vi "SB_OUT.vi"(8 "error in (no error)":errorcluster, 10 "拍攝B讀取條碼":string, 11 "DBLink":string) -> (0 "error out":errorcluster, 2 "待出料":cluster{"條碼A":string, "條碼B":string}, 3 "Workspace: screw_B":cluster{"條碼A":string, "條碼B":string}[](array[cluster]))   [LabVIEW 2019]
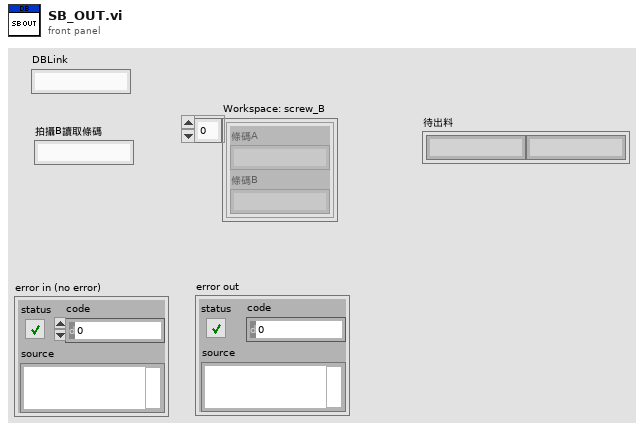
[diagram p1: front panel]
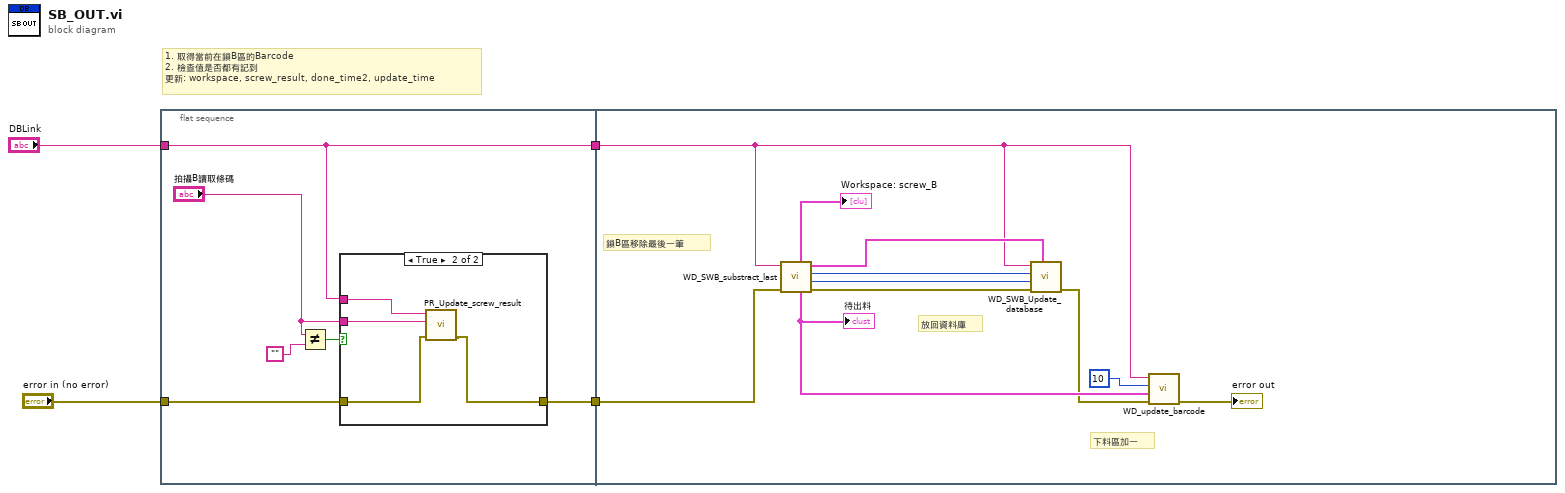
[diagram p0: block diagram]
diagram:
  # "1. 取得當前在鎖B區的Barcode\n2. 檢查值是否都有記到\n更新: workspace, screw_result, done_time2, update_time"
  n1 = flat-sequence {
    tunnel: "DBLink" -> [w6]
    tunnel: "error in (no error)" -> [w8]
    tunnel: [w6] -> w2
    tunnel: [w5] -> w1
    tunnel: w2 -> [w17]
    tunnel: w1 -> [w19]
    frame #0 {
      n2 = Not Equal?(x="拍攝B讀取條碼", y="") -> (x != y?=w9:bool)
      n3 = case shown="True" w9 {
        tunnel: w6 -> [_ w15]
        tunnel: "拍攝B讀取條碼" -> [_ w14]
        tunnel: w8 -> [w11 w13]
        tunnel: [w11 w12] -> w5
        frame False {
        }
        frame True {
          n4 = call "PR_Update_screw_result .vi"("error in (no error)"=w13, "barcode"=w14, "DBlink"=w15) -> ("error out"=w12:errorcluster)  [unwired: 8 in]
        }
      }
    }
    frame #1 {
      # "放回資料庫"
      # "鎖B區移除最後一筆"
      # "下料區加一"
      n5 = call "WD_SWB_substract_last.vi"("error in (no error)"=w19, "DBLink"=w17) -> ("error out"=w25:errorcluster, "站點總數"=w24:i32, "當前料數"=w23:i32, "計算用 array"=w20:cluster{"條碼A":string, "條碼B":string}[], "取出element"=w26:cluster{"條碼A":string, "條碼B":string}, "顯示用array"=→"Workspace: screw_B":cluster{"條碼A":string, "條碼B":string}[])  [unwired: 4 in]
      "待出料" <- w26
      n6 = call "WD_SWB_Update_database.vi"("計算用array"=w20, "error in (no error)"=w25, "站點總數"=w24, "當前料數"=w23, "DBLink"=w17) -> ("error out"=w18:errorcluster)  [unwired: 6 in]
      n7 = call "WD_update_barcode.vi"("error in (no error)"=w18, "Workplace data"=w26, "workplace_id"=i16 10, "DBlink"=w17) -> ("error out"=→"error out":errorcluster)  [unwired: 7 in]
    }
  }
